vi "rqcAlice Delay Line Test (Low Level Example).vi"() -> ()   [LabVIEW 2019]
uses:
  FPGA/Alice/Custom Controls/Phase Modulator/rqcAlice Mod.Config.ctl
  FPGA/Alice/Custom Controls/Main State Machine/rqcAlice DAC Clock Positions.ctl
  Shared/Shared FPGA Lib/Shared Logic/Custom Controls/rqc Random Generator.parameters.ctl
  Shared/Shared FPGA Lib/Shared Logic/Custom Controls/rqc Random Generator.value type.ctl
  Custom Controls/rqcAlice States.ctl
  Shared/Shared Host Lib/rqc ServiceNET/Custom Controls/rqc ServiceNET command.ctl
  Shared/Shared Host Lib/rqc ServiceNET/Alice/Custom Controls/rqcAlice ServiceNET control.ctl
  <vilib>/FPGAPlugInAG/PCIe-7820R/niLvFpga_Open_PCIe-7820R.vi
  <vilib>/rvi/interface/common/dynamic/niFpgaDynamicAddResources.vi
  <vilib>/FPGAPlugInAG/Dynamic/niLvFpga_Close_Dynamic.vi
  <vilib>/rvi/interface/nirviOpenFPGA/nirviOpenFPGA.xnode
  FPGA Bitfiles/rqcAlice FPGA (7820R) v 3.2.0.lvbitx
  <vilib>/rvi/interface/nirviCloseFPGA/nirviCloseFPGA.xnode
panel:
  in  "Tab Control":T1(tab)
  in  "Sync mode":bool caption="«Coax / SD»"
  in  "RndGen.parameters":T2={"value type"=enum."constant", "constant"=0, "num of levels"=4, "levels values"=[0, 0, 0, 0]} caption="Phase modulation value" {"num of levels" min=4 max=4 step=1}
  in  "Delay line min":u32=25000
  in  "Delay line max":u32=27000
  in  "Delay line increment":u32=33 max=200000 step=1
  out "Delay line value scanned":u32=26980
  in  "Modulator config":T4={"mod.on"=9, "mod.off"=1}
  in  "DAC Clock params":T5=[18, 38]
  out "Current State":T6=enum."App.Stop" caption="App current state"
  out "IP Address":string="10.32.64.203"
  out "XY Graph":T7(graph)={"appended array"=[25000.0, 25033.0, 25066.0, 25099.0, 25132.0, 25165.0, 25198.0, 25231.0, 25264.0, 25297.0, 25330.0, 25363.0, 25396.0, 25429.0, 25462.0, 25495.0, 25528.0, 25561.0, 25594.0, 25627.0, 25660.0, 25693.0, 25726.0, 25759.0, 25792.0, 25825.0, 25858.0, 25891.0, 25924.0, 25957.0, 25990.0, 26023.0, 26056.0, 26089.0, 26122.0, 26155.0, 26188.0, 26221.0, 26254.0, 26287.0, 26320.0, 26353.0, 26386.0, 26419.0, 26452.0, 26485.0, 26518.0, 26551.0, 26584.0, 26617.0, 26650.0, 26683.0, 26716.0, 26749.0, 26782.0, 26815.0, 26848.0, 26881.0, 26914.0, 26947.0, 26980.0, 26980.0], "appended array"=[0.0, 0.0, 0.0, 0.0, 0.0, 0.0, 0.0, 0.0, 0.0, 0.0, 0.0, 0.0, 0.0, 0.0, 0.0, 0.0, 0.0, 0.0, 0.0, 0.0, 0.0, 0.0, 0.0, 0.0, 0.0, 0.0, 0.0, 0.0, 0.0, 0.0, 0.0, 0.0, 0.0, 0.0, 0.0, 0.0, 0.0, 0.0, 0.0, 0.0, 0.0, 0.0, 0.0, 0.0, 0.0, 0.0, 0.0, 0.0, 0.0, 0.0, 0.0, 0.0, 0.0, 0.0, 0.0, 0.0, 0.0, 0.0, 0.0, 0.0, 0.0]} caption="Num of Detections vs Delay line value"
  out "error out":errorcluster
  in  "Stop":bool
  out "Connection status":bool
  in  "port":u16=5020
  in  "Attenuation, dB":dbl=10.0 max=40.0
  # "LAN settings:"
  # "«"
  # "»"
  # "Constant"
  # "Random"
  # "Recommended [18]\n[38]"
  # "Recommended mod.on - [9]\nmod.off - [1-2]"
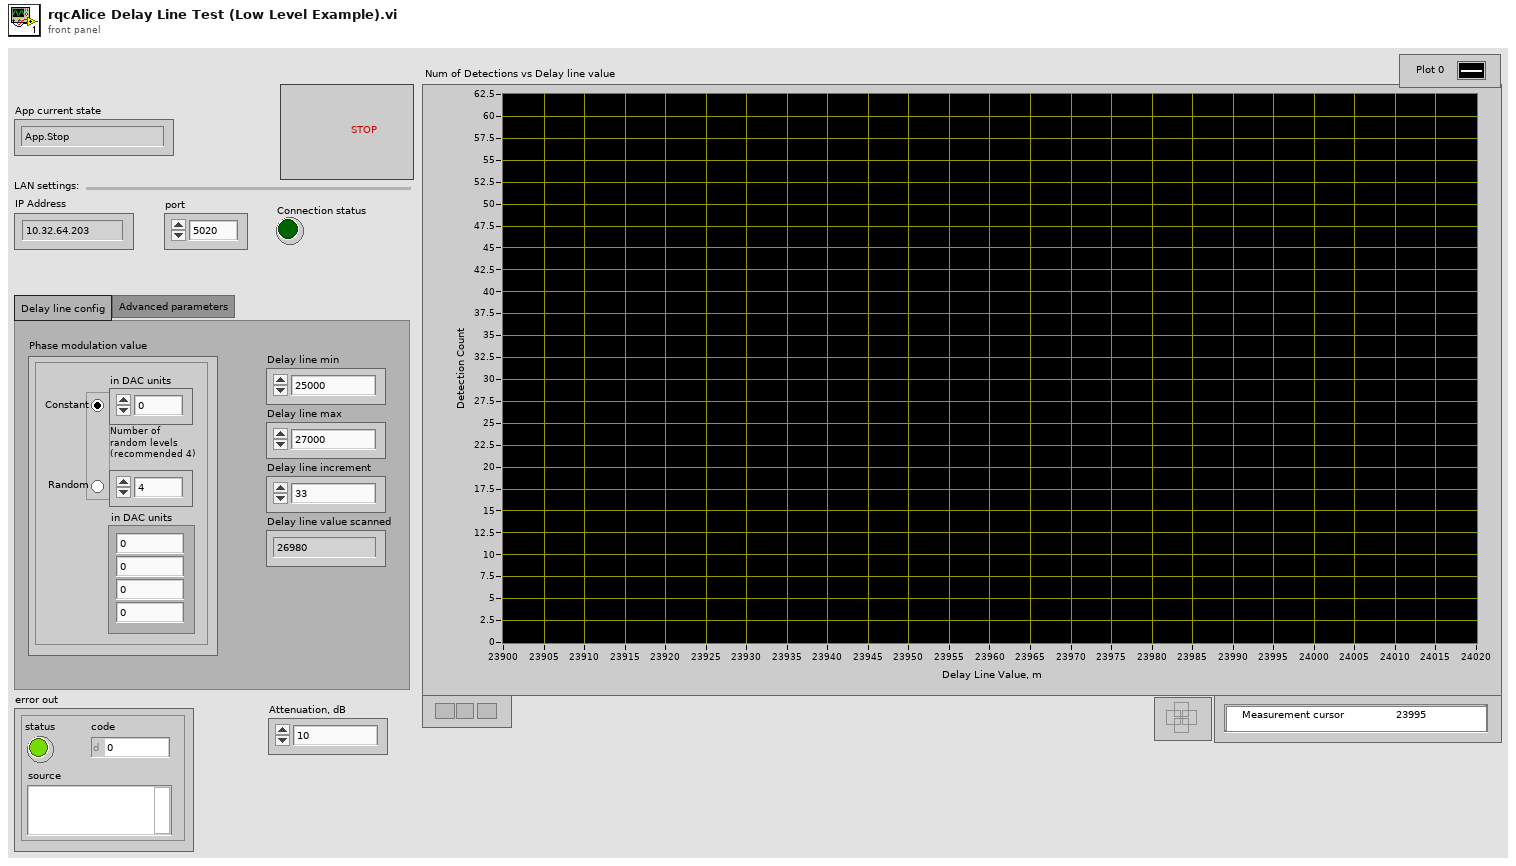
[diagram p1: front panel]
types:
  T1 = enum32{"Delay line config", "Advanced parameters"}
  T2 = typedef "rqc Random Generator.parameters.ctl" = cluster{"value type":T3, "constant":u16, "num of levels":u16, "levels values":u16[]}
  T3 = typedef "rqc Random Generator.value type.ctl" = enum32{"random value", "constant"}
  T4 = typedef "rqcAlice Mod.Config.ctl" = cluster{"mod.on":u8, "mod.off":u8}
  T5 = typedef "rqcAlice DAC Clock Positions.ctl" = u8[]
  T6 = typedef "rqcAlice States.ctl" = enum16{"HW.configure", "HW.meas", "NET.create", "NET.connect", "NET.readCommand", "NET.sendCommand", "NET.readData", "NET.close", "Meas.Start", "Meas.NextStep", "Meas.restart", "Meas.Done", "App.HandleEvent", "App.HandleError", "App.Stop"}
  T7 = cluster{"appended array":dbl[], "appended array":dbl[]}
  T8 = typedef "rqc ServiceNET command.ctl" = enum8{"NONE", "READY", "START", "PING"}
  T9 = typedef "rqcAlice ServiceNET control.ctl" = cluster{"connection ID":refnum<k5>, "port":u16, "connected?":bool}
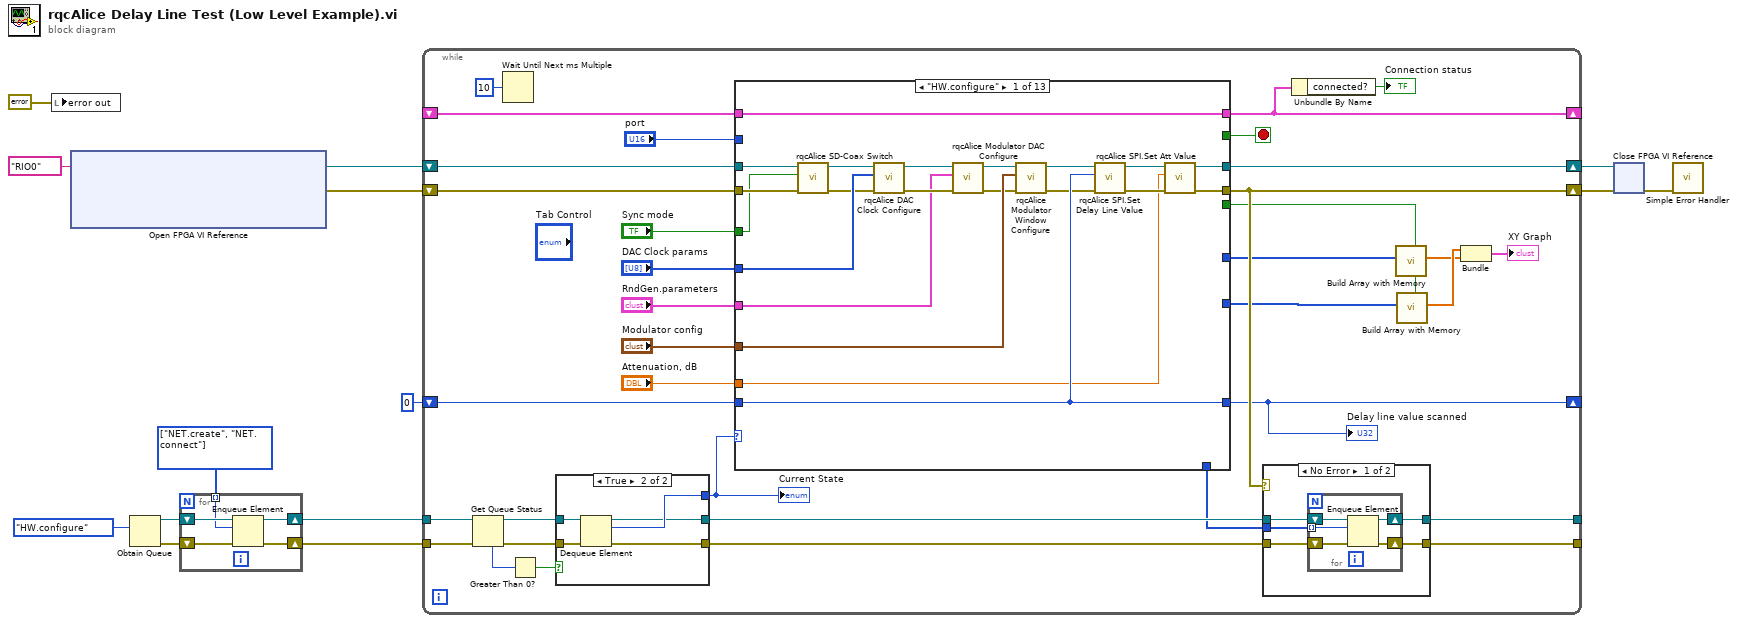
[diagram p0: block diagram]
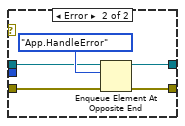
[diagram p2: hidden frame]
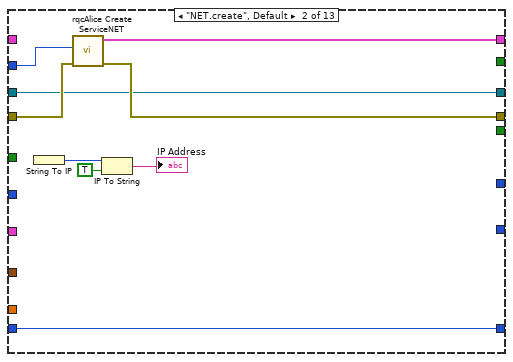
[diagram p3: hidden frame]
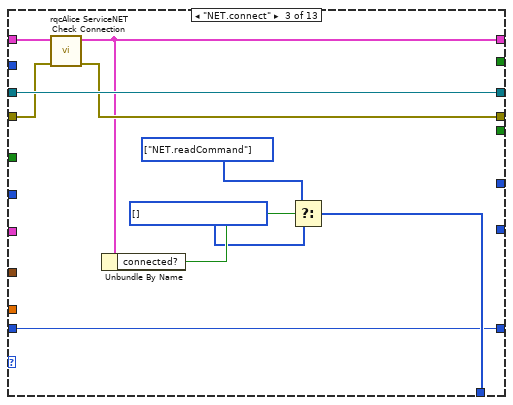
[diagram p4: hidden frame]
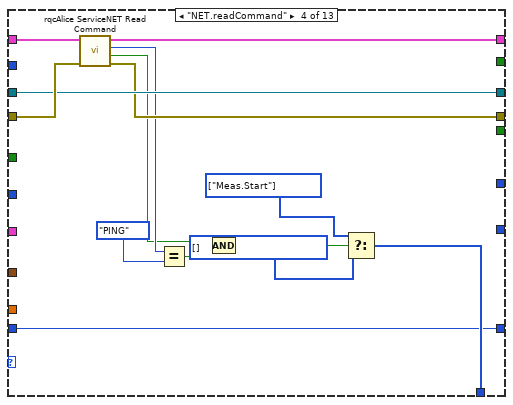
[diagram p5: hidden frame]
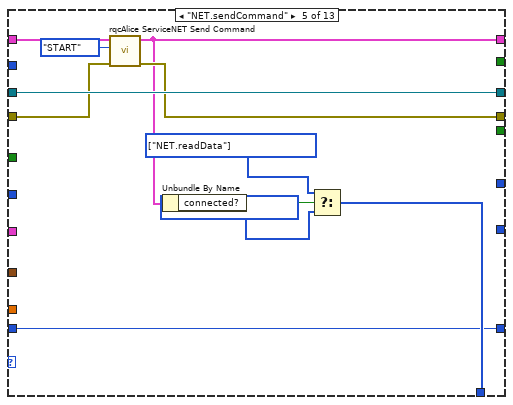
[diagram p6: hidden frame]
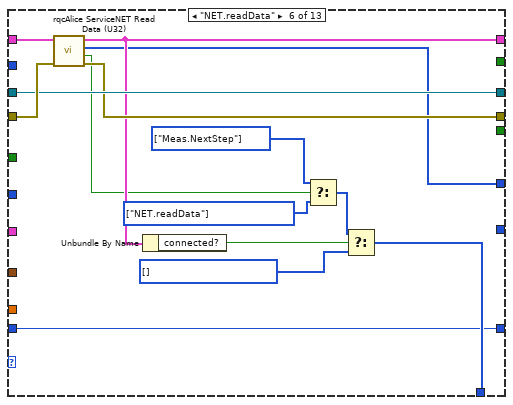
[diagram p7: hidden frame]
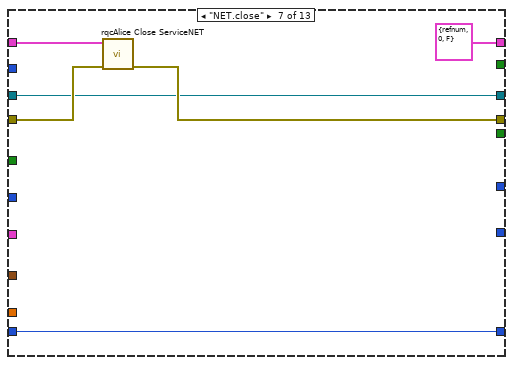
[diagram p8: hidden frame]
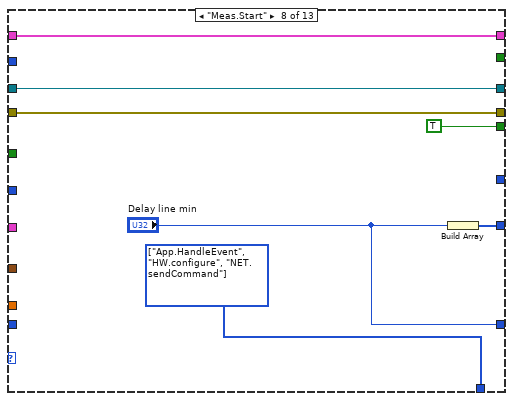
[diagram p9: hidden frame]
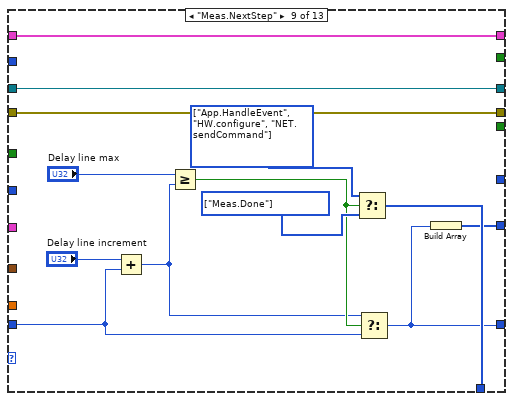
[diagram p10: hidden frame]
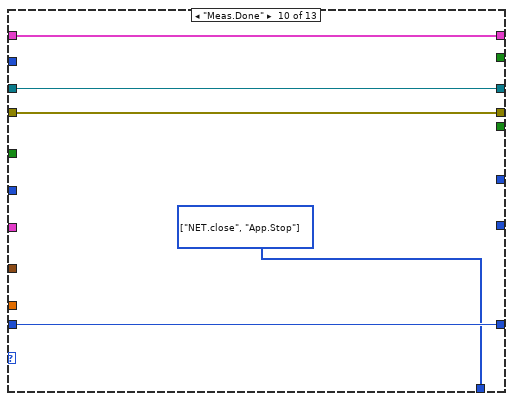
[diagram p11: hidden frame]
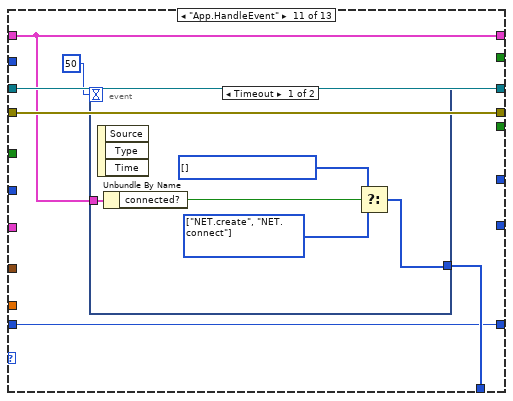
[diagram p12: hidden frame]
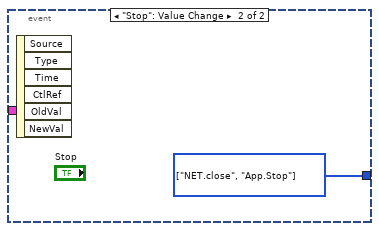
[diagram p13: hidden frame]
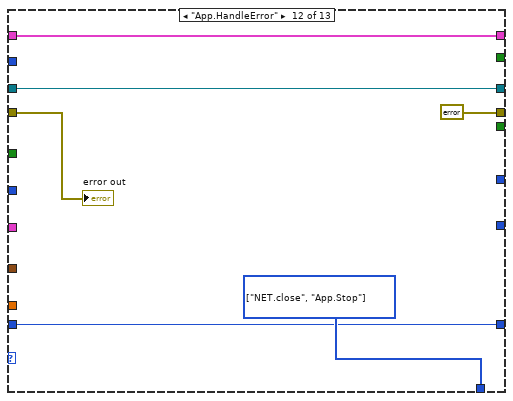
[diagram p14: hidden frame]
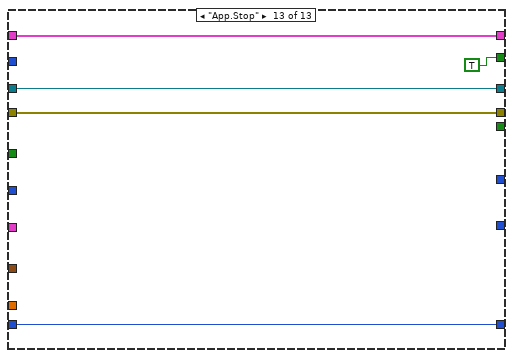
[diagram p15: hidden frame]
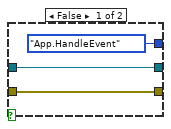
[diagram p16: hidden frame]
diagram:
  w6 = T6[] [enum."NET.create", enum."NET.connect"] items=["HW.configure", "HW.meas", "NET.create", "NET.connect", "NET.readCommand", "NET.sendCommand", "NET.readData", "NET.close", "Meas.Start", "Meas.NextStep", "Meas.restart", "Meas.Done", "App.HandleEvent", "App.HandleError", "App.Stop"]
  n1 = local write "error out"(errorcluster {"status"=FALSE, "code"=0, "source"=""} ("error out")) -> ()
  n2 = xnode "Open FPGA VI Reference"("resource name"=tag "RIO0") -> ("FPGA VI Reference Out"=w13:refnum<k20>, "error out"=w12:errorcluster)  [unwired: 1 in]
  n3 = Obtain Queue(element data type=rqcAlice_States."HW.configure" ("rqcAlice States")) -> (queue out=w8:refnum<queue>, error out=w7:errorcluster)  [unwired: 4 in, 1 out]
  n4 = for {
    shift-right: [w17] -> w5
    shift-left: w8 -> [w19]
    shift-right: [w16] -> w4
    shift-left: w7 -> [w18]
    tunnel: w6 -> [w15] mode=indexing
    n5 = Enqueue Element(queue=w19, element=w15, error in (no error)=w18) -> (queue out=w17:refnum<queue>, error out=w16:errorcluster)  [unwired: 1 in, 1 out]
  }
  n6 = while {
    tunnel: w5 -> [w50]
    shift-right: [w51] -> w11
    shift-left: w13 -> [w54]
    shift-right: [w44] -> w10
    shift-left: w12 -> [w53]
    tunnel: w4 -> [w49]
    tunnel: [w41] -> _
    tunnel: [w40] -> _
    shift-right: [w36] -> _
    shift-left: _ -> [w38]
    shift-right: [w30] -> _
    shift-left: u32 0 ("Delay Line min") -> [w32]
    stop <- w34 stop-if-true
    n7 = Get Queue Status(queue=w50, error in (no error)=w49) -> (queue out=w46:refnum<queue>, error out=w45:errorcluster, # elements in queue=w48:i32)  [unwired: 1 in, 5 out]
    n8 = Wait Until Next ms Multiple(millisecond multiple=u32 10) -> ()  [unwired: 1 out]
    n9 = Greater Than 0?(x=w48) -> (x > 0?=w47:bool)
    n10 = case shown="True" w47 {
      tunnel: w46 -> [w204 w210]
      tunnel: w45 -> [w203 w209]
      tunnel: [rqcAlice_States."App.HandleEvent" ("rqcAlice States") w208] -> w20
      tunnel: [w204 w207] -> w43
      tunnel: [w203 w206] -> w42
      frame False {
      }
      frame True {
        n11 = Dequeue Element(queue=w210, error in (no error)=w209) -> (queue out=w207:refnum<queue>, element=w208:T6, error out=w206:errorcluster)  [unwired: 1 in, 1 out]
      }
    }
    "Current State" <- w20
    n12 = case shown="\"HW.configure\"" w20 {
      tunnel: w54 -> [w87 w96 w109 w120 w134 w146 w150 w160 w173 w178 w185 w196 w201]
      tunnel: w53 -> [w86 w98 w107 w122 w132 w147 w153 w159 w172 w177 w184 w195 w200]
      tunnel: "Modulator config" -> [w90 _ _ _ _ _ _ _ _ _ _ _ _]
      tunnel: [w78 w96 w109 w120 w134 w146 w150 w160 w173 w178 w185 w196 w201] -> w51
      tunnel: [w76 w97 w106 w119 w131 w145 w152 w159 w172 w177 w184 errorcluster {"status"=FALSE, "code"=0, "source"=""} ("error out") w200] -> w44
      tunnel: [_ _ w102 w111 w125 w137 _ w158 w168 w175 w181 w193 _] -> w39
      tunnel: [w89 w99 w105 w121 w129 w144 T9 {"connection ID"=refnum, "port"=0, "connected?"=FALSE} ("rqcAlice ServiceNET out") w161 w174 w179 w182 w197 w199] -> w36
      tunnel: w38 -> [w89 _ w108 w123 w133 w148 w154 w161 w174 w179 w182 w197 w199]
      tunnel: "port" -> [_ w95 _ _ _ _ _ _ _ _ _ _ _]
      tunnel: [_ _ _ _ _ _ _ _ _ _ _ _ TRUE] -> w34
      tunnel: w32 -> [w81 w94 w100 w110 w124 w136 w149 _ w164 w176 w180 w192 w198]
      tunnel: [w81 w94 w100 w110 w124 w136 w149 "Delay line min" w163 w176 w180 w192 w198] -> w30
      tunnel: [_ _ _ _ _ w135 _ _ _ _ _ _ _] -> w31
      tunnel: [_ _ _ _ _ _ _ w155 w162 _ _ _ _] -> w29
      tunnel: [_ _ _ _ _ _ _ TRUE _ _ _ _ _] -> w28
      tunnel: "DAC Clock params" -> [w88 _ _ _ _ _ _ _ _ _ _ _ _]
      tunnel: "RndGen.parameters" -> [w70 _ _ _ _ _ _ _ _ _ _ _ _]
      tunnel: "Sync mode" -> [w83 _ _ _ _ _ _ _ _ _ _ _ _]
      tunnel: "Attenuation, dB" -> [w75 _ _ _ _ _ _ _ _ _ _ _ _]
      frame "HW.configure" {
        n13 = call "rqcAlice SD-Coax Switch.vi"("error in"=w86, "SD/Coax Select"=w83, "Alice FPGA Reference In"=w87) -> ("error out"=w84:errorcluster, "Alice FPGA Reference Out"=w85:refnum<k20>)  [unwired: 7 in]
        n14 = call "rqcAlice DAC Clock Configure.vi"("error in"=w84, "DAC Clock params"=w88, "Alice FPGA Reference In"=w85) -> ("error out"=w71:errorcluster, "Alice FPGA Reference Out"=w74:refnum<k20>)  [unwired: 7 in]
        n15 = call "rqcAlice Modulator DAC Configure.vi"("error in"=w71, "RndGen.parameters"=w70, "Alice FPGA Reference In"=w74) -> ("error out"=w72:errorcluster, "Alice FPGA Reference Out"=w73:refnum<k20>)  [unwired: 7 in]
        n16 = call "rqcAlice Modulator Window Configure.vi"("error in"=w72, "Modulator config"=w90, "Alice FPGA Reference In"=w73) -> ("error out"=w80:errorcluster, "Alice FPGA Reference Out"=w82:refnum<k20>)  [unwired: 7 in]
        n17 = call "rqcAlice SPI.Set Delay Line Value.vi"("error in"=w80, "Delay Line Value"=w81, "Alice FPGA Reference In"=w82) -> ("error out"=w77:errorcluster, "Alice FPGA Reference Out"=w79:refnum<k20>)  [unwired: 7 in]
        n18 = call "rqcAlice SPI.Set Att Value.vi"("error in"=w77, "Attenuation, dB"=w75, "Alice FPGA Reference In"=w79) -> ("error out"=w76:errorcluster, "Alice FPGA Reference Out"=w78:refnum<k20>)  [unwired: 7 in]
      }
      frame "NET.create", Default {
        n19 = String To IP() -> (0:w92:u32)  [unwired: 1 in]
        n20 = call "rqcAlice Create ServiceNET.vi"("error in"=w98, "port"=w95) -> ("error out"=w97:errorcluster, "rqcAlice ServiceNET control"=w99:T9)  [unwired: 8 in]
        n21 = IP To String(1:TRUE ("dot notation? (F)"), 2:w92) -> (0:→"IP Address":string)
      }
      frame "NET.connect" {
        w101 = T6[] [] items=["HW.configure", "HW.meas", "NET.create", "NET.connect", "NET.readCommand", "NET.sendCommand", "NET.readData", "NET.close", "Meas.Start", "Meas.NextStep", "Meas.restart", "Meas.Done", "App.HandleEvent", "App.HandleError", "App.Stop"] ("f")
        w103 = T6[] [enum."NET.readCommand"] items=["HW.configure", "HW.meas", "NET.create", "NET.connect", "NET.readCommand", "NET.sendCommand", "NET.readData", "NET.close", "Meas.Start", "Meas.NextStep", "Meas.restart", "Meas.Done", "App.HandleEvent", "App.HandleError", "App.Stop"]
        n22 = call "rqcAlice ServiceNET Check Connection.vi"("error in"=w107, "rqcAlice ServiceNET in"=w108) -> ("error out"=w106:errorcluster, "rqcAlice ServiceNET out"=w105:T9)  [unwired: 8 in]
        n23 = Unbundle By Name(w105) -> ("connected?"=w104:bool)
        n24 = Select(t=w103, s=w104, f=w101) -> (s? t:f=w102:T6[])
      }
      frame "NET.readCommand" {
        w112 = T6[] [] items=["HW.configure", "HW.meas", "NET.create", "NET.connect", "NET.readCommand", "NET.sendCommand", "NET.readData", "NET.close", "Meas.Start", "Meas.NextStep", "Meas.restart", "Meas.Done", "App.HandleEvent", "App.HandleError", "App.Stop"] ("f")
        w113 = T6[] [enum."Meas.Start"] items=["HW.configure", "HW.meas", "NET.create", "NET.connect", "NET.readCommand", "NET.sendCommand", "NET.readData", "NET.close", "Meas.Start", "Meas.NextStep", "Meas.restart", "Meas.Done", "App.HandleEvent", "App.HandleError", "App.Stop"] ("f")
        n25 = call "rqcAlice ServiceNET Read Command.vi"("error in"=w122, "rqcAlice ServiceNET in"=w123) -> ("error out"=w119:errorcluster, "cmd valid"=w115:bool, "command"=w117:T8, "rqcAlice ServiceNET out"=w121:T9)  [unwired: 6 in]
        n26 = Equal?(x=w117, y=rqc_ServiceNET_command."PING" ("command")) -> (x = y?=w116:bool)
        n27 = Compound Arithmetic op=AND(w115, w116) -> (w114:bool)
        n28 = Select(t=w113, s=w114, f=w112) -> (s? t:f=w111:T6[])
      }
      frame "NET.sendCommand" {
        w126 = T6[] [] items=["HW.configure", "HW.meas", "NET.create", "NET.connect", "NET.readCommand", "NET.sendCommand", "NET.readData", "NET.close", "Meas.Start", "Meas.NextStep", "Meas.restart", "Meas.Done", "App.HandleEvent", "App.HandleError", "App.Stop"] ("f")
        w127 = T6[] [enum."NET.readData"] items=["HW.configure", "HW.meas", "NET.create", "NET.connect", "NET.readCommand", "NET.sendCommand", "NET.readData", "NET.close", "Meas.Start", "Meas.NextStep", "Meas.restart", "Meas.Done", "App.HandleEvent", "App.HandleError", "App.Stop"] ("f")
        n29 = call "rqcAlice ServiceNET Send Command.vi"("error in"=w132, "command"=rqc_ServiceNET_command."START", "rqcAlice ServiceNET in"=w133) -> ("error out"=w131:errorcluster, "rqcAlice ServiceNET out"=w129:T9)  [unwired: 7 in]
        n30 = Unbundle By Name(w129) -> ("connected?"=w128:bool)
        n31 = Select(t=w127, s=w128, f=w126) -> (s? t:f=w125:T6[])
      }
      frame "NET.readData" {
        w138 = T6[] [] items=["HW.configure", "HW.meas", "NET.create", "NET.connect", "NET.readCommand", "NET.sendCommand", "NET.readData", "NET.close", "Meas.Start", "Meas.NextStep", "Meas.restart", "Meas.Done", "App.HandleEvent", "App.HandleError", "App.Stop"] ("f")
        w143 = T6[] [enum."Meas.NextStep"] items=["HW.configure", "HW.meas", "NET.create", "NET.connect", "NET.readCommand", "NET.sendCommand", "NET.readData", "NET.close", "Meas.Start", "Meas.NextStep", "Meas.restart", "Meas.Done", "App.HandleEvent", "App.HandleError", "App.Stop"] ("t")
        w141 = T6[] [enum."NET.readData"] items=["HW.configure", "HW.meas", "NET.create", "NET.connect", "NET.readCommand", "NET.sendCommand", "NET.readData", "NET.close", "Meas.Start", "Meas.NextStep", "Meas.restart", "Meas.Done", "App.HandleEvent", "App.HandleError", "App.Stop"] ("f")
        n32 = call "rqcAlice ServiceNET Read Data (U32).vi"("error in"=w147, "rqcAlice ServiceNET in"=w148) -> ("error out"=w145:errorcluster, "data valid"=w142:bool, "data"=w135:u32[], "rqcAlice ServiceNET out"=w144:T9)  [unwired: 6 in]
        n33 = Unbundle By Name(w144) -> ("connected?"=w140:bool)
        n34 = Select(t=w143, s=w142, f=w141) -> (s? t:f=w139:T6[])
        n35 = Select(t=w139, s=w140, f=w138) -> (s? t:f=w137:T6[])
      }
      frame "NET.close" {
        n36 = call "rqcAlice Close ServiceNET.vi"("error in"=w153, "rqcAlice ServiceNET in"=w154) -> ("error out"=w152:errorcluster)  [unwired: 9 in]
      }
      frame "Meas.Start" {
        w158 = T6[] [enum."App.HandleEvent", enum."HW.configure", enum."NET.sendCommand"] items=["HW.configure", "HW.meas", "NET.create", "NET.connect", "NET.readCommand", "NET.sendCommand", "NET.readData", "NET.close", "Meas.Start", "Meas.NextStep", "Meas.restart", "Meas.Done", "App.HandleEvent", "App.HandleError", "App.Stop"] ("f")
        n37 = Build Array("Delay line min") -> (w155:u32[])
      }
      frame "Meas.NextStep" {
        w167 = T6[] [enum."Meas.Done"] items=["HW.configure", "HW.meas", "NET.create", "NET.connect", "NET.readCommand", "NET.sendCommand", "NET.readData", "NET.close", "Meas.Start", "Meas.NextStep", "Meas.restart", "Meas.Done", "App.HandleEvent", "App.HandleError", "App.Stop"] ("f")
        w169 = T6[] [enum."App.HandleEvent", enum."HW.configure", enum."NET.sendCommand"] items=["HW.configure", "HW.meas", "NET.create", "NET.connect", "NET.readCommand", "NET.sendCommand", "NET.readData", "NET.close", "Meas.Start", "Meas.NextStep", "Meas.restart", "Meas.Done", "App.HandleEvent", "App.HandleError", "App.Stop"] ("f")
        n38 = Add(x="Delay line increment", y=w164) -> (x+y=w165:u32)
        n39 = Greater Or Equal?(x="Delay line max", y=w165) -> (x >= y?=w166:bool)
        n40 = Select(t=w169, s=w166, f=w167) -> (s? t:f=w168:T6[])
        n41 = Select(t=w165, s=w166, f=w164) -> (s? t:f=w163:u32)
        n42 = Build Array(w163) -> (w162:u32[])
      }
      frame "Meas.Done" {
        w175 = T6[] [enum."NET.close", enum."App.Stop"] items=["HW.configure", "HW.meas", "NET.create", "NET.connect", "NET.readCommand", "NET.sendCommand", "NET.readData", "NET.close", "Meas.Start", "Meas.NextStep", "Meas.restart", "Meas.Done", "App.HandleEvent", "App.HandleError", "App.Stop"] ("f")
      }
      frame "App.HandleEvent" {
        n43 = event shown="[0] Timeout" {
          selector: _ -> [_ _]
          dyn-events: _ -> [_ _]
          timeout: 50 -> [_ _]
          tunnel: w182 -> [w190 _]
          tunnel: [w186 w191] -> w181
          event Timeout {
            w187 = T6[] [enum."NET.create", enum."NET.connect"] items=["HW.configure", "HW.meas", "NET.create", "NET.connect", "NET.readCommand", "NET.sendCommand", "NET.readData", "NET.close", "Meas.Start", "Meas.NextStep", "Meas.restart", "Meas.Done", "App.HandleEvent", "App.HandleError", "App.Stop"]
            w188 = T6[] [] items=["HW.configure", "HW.meas", "NET.create", "NET.connect", "NET.readCommand", "NET.sendCommand", "NET.readData", "NET.close", "Meas.Start", "Meas.NextStep", "Meas.restart", "Meas.Done", "App.HandleEvent", "App.HandleError", "App.Stop"]
            n44 = event-data() -> ()  [unwired: 1 in, 3 out]
            n45 = Unbundle By Name(w190) -> ("connected?"=w189:bool)
            n46 = Select(t=w188, s=w189, f=w187) -> (s? t:f=w186:T6[])
          }
          event "Stop": Value Change {
            w191 = T6[] [enum."NET.close", enum."App.Stop"] items=["HW.configure", "HW.meas", "NET.create", "NET.connect", "NET.readCommand", "NET.sendCommand", "NET.readData", "NET.close", "Meas.Start", "Meas.NextStep", "Meas.restart", "Meas.Done", "App.HandleEvent", "App.HandleError", "App.Stop"]
            n47 = event-data() -> ()  [unwired: 1 in, 6 out]
          }
        }
      }
      frame "App.HandleError" {
        w193 = T6[] [enum."NET.close", enum."App.Stop"] items=["HW.configure", "HW.meas", "NET.create", "NET.connect", "NET.readCommand", "NET.sendCommand", "NET.readData", "NET.close", "Meas.Start", "Meas.NextStep", "Meas.restart", "Meas.Done", "App.HandleEvent", "App.HandleError", "App.Stop"] ("f")
        "error out" <- w195
      }
      frame "App.Stop" {
      }
    }
    "Delay line value scanned" <- w30
    n48 = case shown="No Error" w44 {
      tunnel: w43 -> [w59 w68]
      tunnel: w42 -> [w58 w66]
      tunnel: [w57 w67] -> w41
      tunnel: [w56 w65] -> w40
      tunnel: w39 -> [w55 _]
      frame No Error {
        n49 = for {
          shift-right: [w62] -> w57
          shift-left: w59 -> [w64]
          shift-right: [w61] -> w56
          shift-left: w58 -> [w63]
          tunnel: w55 -> [w60] mode=indexing
          n50 = Enqueue Element(queue=w64, element=w60, error in (no error)=w63) -> (queue out=w62:refnum<queue>, error out=w61:errorcluster)  [unwired: 1 in, 1 out]
        }
      }
      frame Error {
        n51 = Enqueue Element At Opposite End(queue=w68, element=rqcAlice_States."App.HandleError" ("rqcAlice States"), error in (no error)=w66) -> (queue out=w67:refnum<queue>, error out=w65:errorcluster)  [unwired: 1 in, 1 out]
      }
    }
    n52 = Unbundle By Name(w36) -> ("connected?"=→"Connection status":bool)
    n53 = call "Build Array with Memory.vi"("reset"=w28, "new array"=w31) -> ("appended array"=w25:dbl[])  [unwired: 9 in]
    n54 = call "Build Array with Memory.vi"("reset"=w28, "new array"=w29) -> ("appended array"=w26:dbl[])  [unwired: 9 in]
    n55 = Bundle("appended array"=w26, "appended array"=w25) -> (→"XY Graph":T7)  [unwired: 1 in]
  }
  n56 = xnode "Close FPGA VI Reference"("FPGA VI Reference In"=w11, "error in"=w10) -> ("error out"=w3:errorcluster)
  n57 = call <vilib>:"Simple Error Handler.vi"("error in (no error)"=w3) -> ()  [unwired: 4 in, 5 out]
